vi "GetServerVIName.vi"(1 "Baxter":T1) -> (0 "vi name":string)   [LabVIEW 2013]
uses:
  _ROSControl.ctl
  _ROSDirection.ctl
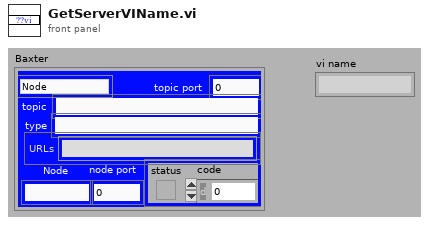
[diagram p1: front panel]
types:
  T1 = typedef "_ROSControl.ctl" = cluster{"topic port":u16, "Node":string, "topic":string, "type":string, "node port":u32, "error ":errorcluster, "Direction":T2, "APIs":string[]}
  T2 = typedef "_ROSDirection.ctl" = enum16{"Node", "Publisher", "Subscriber", "Service Client"}
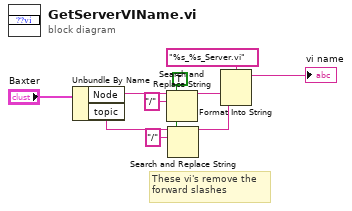
[diagram p0: block diagram]
diagram:
  w4 = TRUE ("replace all? (F)")
  # "These vi's remove the \nforward slashes"
  n1 = Unbundle By Name("Baxter") -> ("Node"=w8:string, "topic"=w9:string)
  n2 = Search and Replace String(replace all?=w4, input string=w8, search string="/" ("regular expression")) -> (result string=w2:string)  [unwired: 5 in, 3 out]
  n3 = Search and Replace String(replace all?=w4, input string=w9, search string="/" ("regular expression")) -> (result string=w5:string)  [unwired: 5 in, 3 out]
  n4 = Format Into String(format string="%s_%s_Server.vi", w2, w5) -> (resulting string=→"vi name":string)  [unwired: 2 in, 1 out]
